vi "raceCondition.vi"() -> ()   [LabVIEW 2020]
panel:
  out "Total":i32
  out "L2":i32
  out "L1":i32
  in  "stop":bool
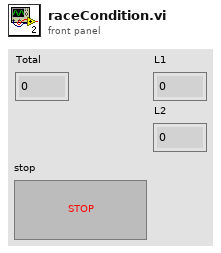
[diagram p1: front panel]
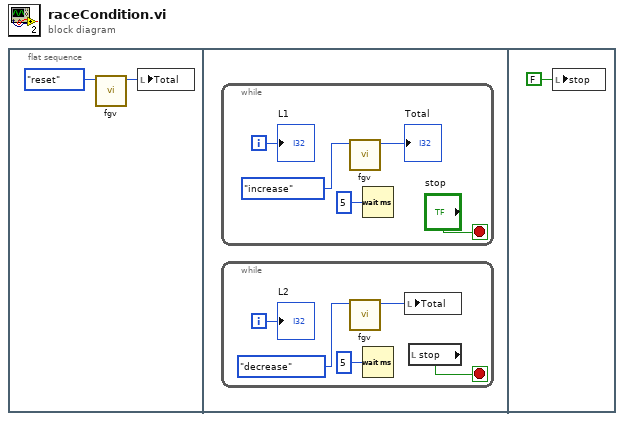
[diagram p0: block diagram]
diagram:
  n1 = flat-sequence {
    frame #0 {
      n2 = call "fgv.vi"("Function"=enum16{"reset", "increase", "decrease"}."reset") -> ("Total"=w2:i32)  [unwired: 10 in]
      n3 = local write "Total"(w2) -> ()
    }
    frame #1 {
      n4 = while {
        i -> [w11]
        stop <- "stop" stop-if-true
        n5 = call "fgv.vi"("Function"=enum16{"reset", "increase", "decrease"}."increase") -> ("Total"=→"Total":i32)  [unwired: 10 in]
        n6 = Wait (ms)(milliseconds to wait=u32 5) -> ()  [unwired: 1 out]
        "L1" <- w11
      }
      n7 = while {
        i -> [w6]
        stop <- w7 stop-if-true
        n8 = call "fgv.vi"("Function"=enum16{"reset", "increase", "decrease"}."decrease") -> ("Total"=w4:i32)  [unwired: 10 in]
        n9 = Wait (ms)(milliseconds to wait=u32 5) -> ()  [unwired: 1 out]
        n10 = local write "Total"(w4) -> ()
        n11 = local read "stop"() -> (w7:bool)
        "L2" <- w6
      }
    }
    frame #2 {
      n12 = local write "stop"(FALSE ("stop")) -> ()
    }
  }
